vi "Run Tests - When Theory Provided - Sets Control Data.vi"() -> ()   [LabVIEW 2017, in "LVUnit Test Executor.Tests.lvlib"]
uses:
  LVUnit Test Executor.Tests.lvlib
  LVUnit Test Executor/LVUnit Test Executor.lvclass
  Test Outcome.ctl
  LVUnit Test Case/LVUnit Test Case.lvclass
  C:/Users/pasca/source/repos/lvunit/Test Case/Test Case.lvclass
  LVUnit Test Case/LVUnit Test Case.lvclass/LVUnit Test Case.ctl
  Test Result/Test Result.lvclass/Test Result.ctl
  69cb7921-841e-4c9d-a7cd-5bddb525d99d.vi
  LVUnit Test Case/Set JSON Data.vi
  Test Result/Get Outcome.vi
  Fake Theory.vi
  Constraint/IsEqual/Create.vi
  Constraint/IsEqual/IsEqual.lvclass
  Test Case/Test Case.lvclass
  Test Result/Test Result.lvclass
panel:
  out "error out":errorcluster
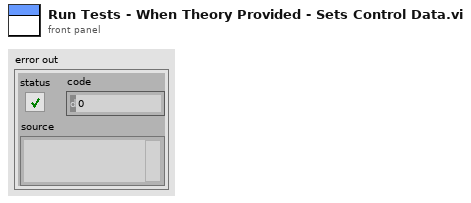
[diagram p1: front panel]
types:
  T1 = typedef "Test Outcome.ctl" = enum16{"None", "Passed", "Failed"}
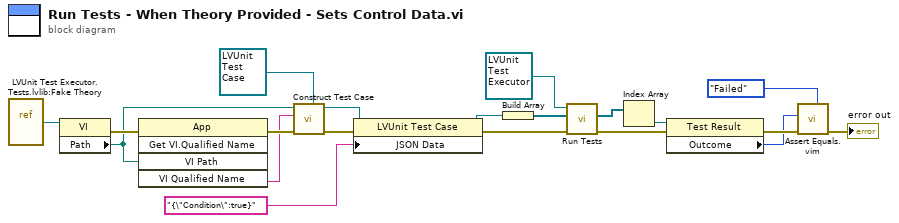
[diagram p0: block diagram]
diagram:
  n1 = vi-ref "LVUnit Test Executor.Tests.lvlib:Fake Theory.vi"() -> (w20:refnum<vi>)
  n2 = property class="VI"(reference=w20) -> (error out=w19:errorcluster, "Path"=w18:path)  [unwired: 1 in, 1 out]
  n3 = invoke class="App" method="Get VI.Qualified Name"(error in=w19, "VI Path"=w18) -> (error out=w17:errorcluster, "VI Qualified Name"=w16:string)  [unwired: 3 in, 3 out]
  n4 = call "Construct Test Case.vi"("Test Case in"=refnum<class "LVUnit Test Case.lvclass"> refnum ("LVUnit Test Case"), "error in (no error)"=w17, "Qualified Name"=w16, "Path"=w18) -> ("error out"=w15:errorcluster, "Test Case out"=w8:refnum<class "LVUnit Test Case.lvclass">)  [unwired: 6 in]
  n5 = property class="LVUnit Test Case"(reference=w8, error in=w15, "JSON Data"="{\"Condition\":true}") -> (reference out=w7:refnum<class "LVUnit Test Case.lvclass">, error out=w9:errorcluster)
  n6 = Build Array(w7) -> (w14:refnum<class "LVUnit Test Case.lvclass">[])
  n7 = call-dynamic "Run Tests.vi"("error in (no error)"=w9, "Test Cases"=w14, "LVUnit Test Executor in"=refnum<class "LVUnit Test Executor.lvclass"> refnum ("LVUnit Test Executor")) -> ("error out"=w12:errorcluster, "Test Results"=w11:refnum<class "Test Result.lvclass">[])  [unwired: 6 in, 1 out]
  n8 = Index Array(array=w11) -> (element=w10:refnum<class "Test Result.lvclass">)  [unwired: 1 in]
  n9 = property class="Test Result"(reference=w10, error in=w12) -> (error out=w6:errorcluster, "Outcome"=w5:T1)  [unwired: 1 out]
  n10 = call "Assert Equals.vim"("Expected"=Test_Outcome."Failed" ("Outcome"), "error in (no error)"=w6, "Actual"=w5) -> ("error out"=→"error out":errorcluster)  [unwired: 8 in]
